vi "simulation analysis.vi"() -> ()   [LabVIEW 2009]
uses:
  subVIs/simulate (multiple).vi
  <vilib>/Utility/file.llb/Read From Spreadsheet File (I64).vi
  <vilib>/Analysis/NI_AALBase.lvlib
panel:
  out "y axis 2":dbl
  out "x axis 2":dbl
  out "x axis":dbl
  out "y axis":dbl
  out "output cluster":cluster{dbl[], "Best Linear Fit":dbl[]}[](graph)
  out "matches":i16[][](array[numeric])
  in  "source data folder(s)":cluster{"file path":path, "depth":i32}[](array[cluster])
  in  "estimated team value data":path
  # "blue score"
  # "red score"
  # "est blue"
  # "est red"
  # "red"
  # "blue"
  # "3"
  # "1"
  # "2"
  # "3"
  # "1"
  # "2"
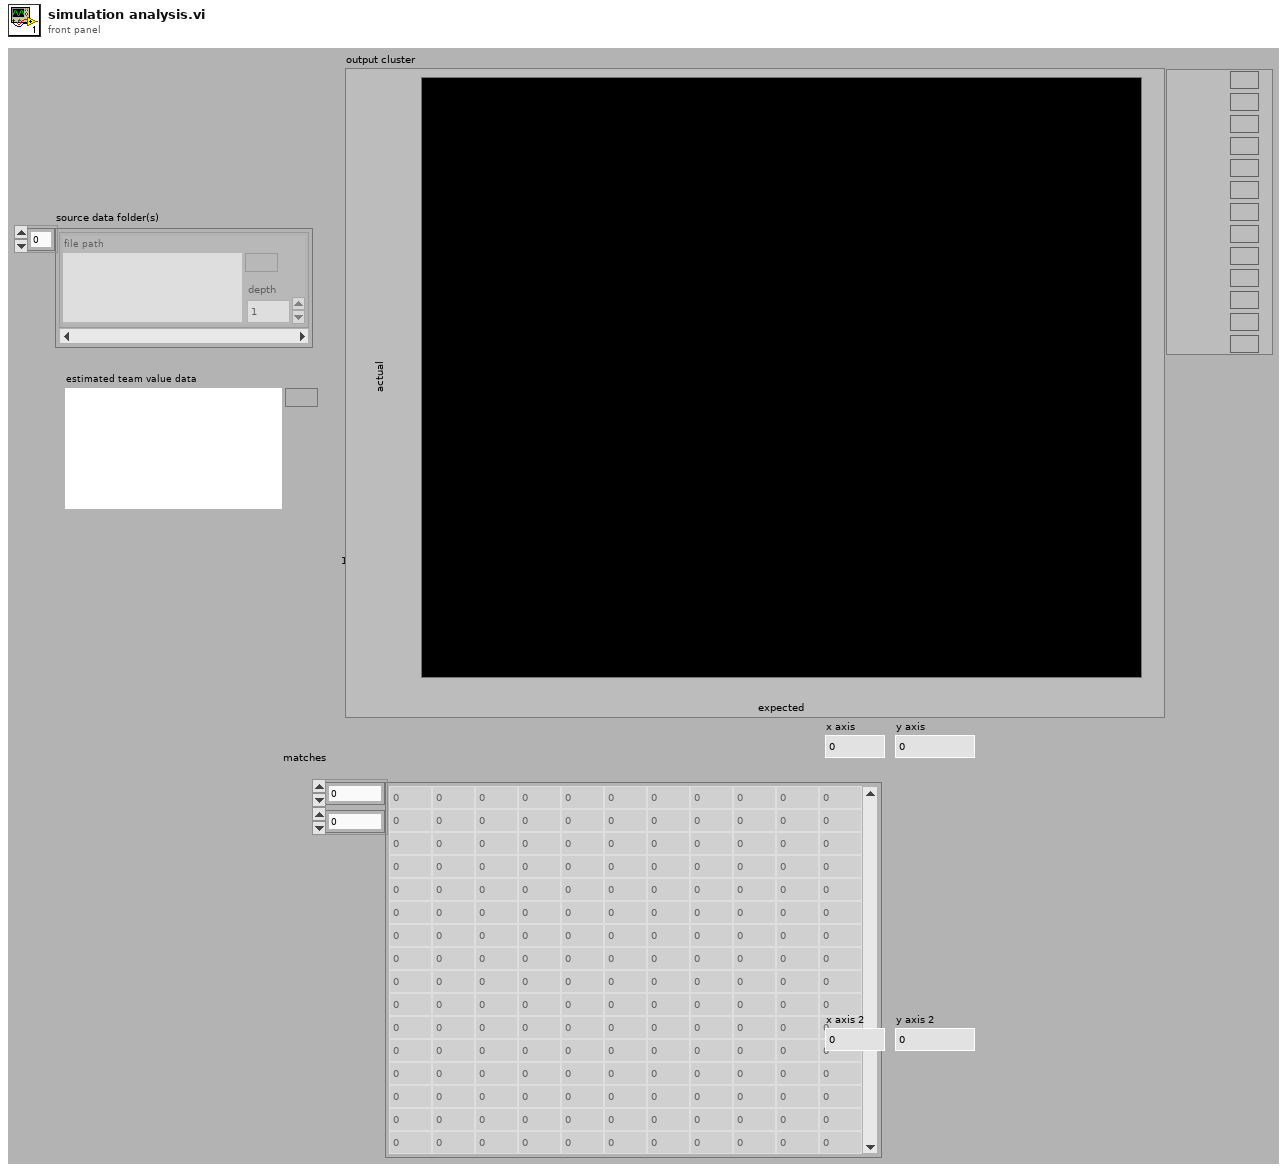
[diagram p1: front panel]
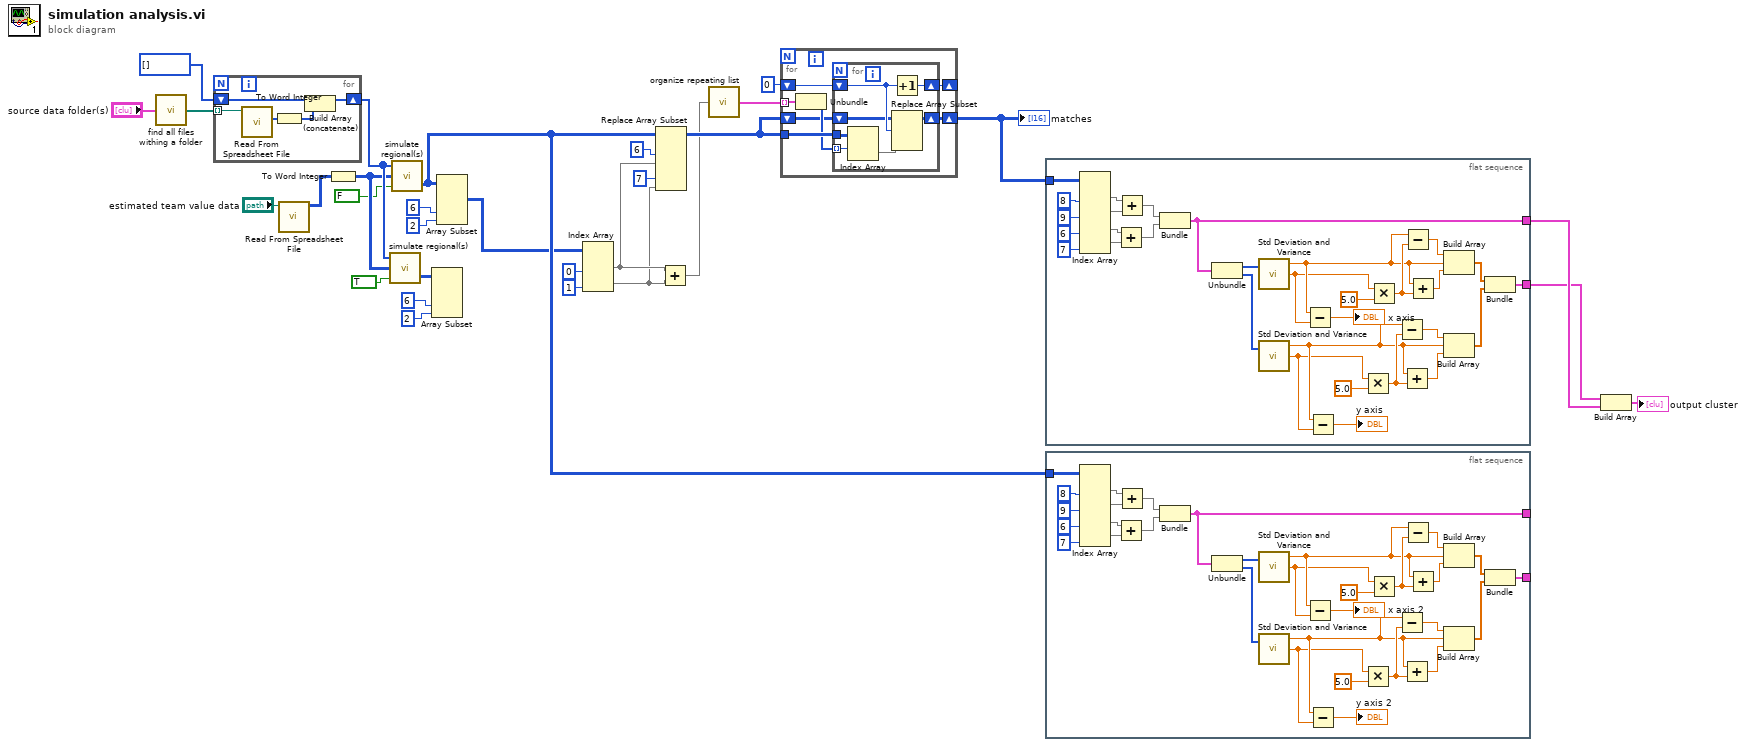
[diagram p0: block diagram]
diagram:
  n1 = call "find all files withing a folder.vi"("folders"="source data folder(s)") -> ("paths"=w28:path[])  [unwired: 1 out]
  n2 = for {
    shift-right: [w33] -> w21
    shift-left: i16[] [] -> [w31]
    tunnel: w28 -> [w34] mode=indexing
    n3 = call-poly <vilib>:"Read From Spreadsheet File.vi"("file path (dialog if empty)"=w34) -> ("first row"=w35:i64[])  [unwired: 6 in, 4 out]
    n4 = To Word Integer(number=w35) -> (16bit integer=w32:i16[])
    n5 = Build Array (concatenate)(w31, w32) -> (w33:i16[])
  }
  n6 = call-poly <vilib>:"Read From Spreadsheet File.vi"("file path (dialog if empty)"="estimated team value data") -> ("all rows"=w23:i64[][])  [unwired: 6 in, 4 out]
  n7 = To Word Integer(number=w23) -> (16bit integer=w20:i16[][])
  n8 = call-poly "simulate regional(s).vi"("liability?  (benefit)"=TRUE, "estimated values"=w20, "source data"=w21) -> ("Array"=w13:i16[][])  [unwired: 1 out]
  n9 = call-poly "simulate regional(s).vi"("liability?  (benefit)"=FALSE, "estimated values"=w20, "source data"=w21) -> ("Array"=w5:i16[][])  [unwired: 1 out]
  n10 = Array Subset(array=w13, index (col)=6 ("disabled index (col)"), length (col)=2 ("disabled index (col)")) -> ()  [unwired: 2 in, 1 out]
  n11 = Array Subset(array=w5, index (col)=6 ("disabled index (col)"), length (col)=2 ("disabled index (col)")) -> (w1:i16[][])  [unwired: 2 in]
  n12 = Index Array(array=w1, index (col) #1=0 ("disabled index (col)"), index (col) #2=1 ("index (col)")) -> (element #1=w8:i16[], element #2=w7:i16[])  [unwired: 2 in]
  n13 = Replace Array Subset(array=w5, new element #1=w8, index (col) #1=6 ("disabled index (col)"), new element #2=w7, index (col) #2=7 ("index (col)")) -> (w18:i16[][])  [unwired: 2 in]
  n14 = Add(x=w8, y=w7) -> (x+y=w6:i16[])
  n15 = call "organize repeating list.vi"("Array in"=w6) -> ("Array out"=w27:cluster{i16, i32[]}[])
  n16 = for {
    tunnel: w27 -> [w42] mode=indexing
    tunnel: w18 -> [w41]
    shift-right: [w38] -> w24
    shift-left: w18 -> [w37]
    shift-right: [w36] -> _
    shift-left: 0 -> [w39]
    n17 = Unbundle(w42) -> (w40:i32[])  [unwired: 1 out]
    n18 = for {
      tunnel: w41 -> [w49]
      tunnel: w40 -> [w48] mode=indexing
      shift-right: [w47] -> w36
      shift-left: w39 -> [w45]
      shift-right: [w44] -> w38
      shift-left: w37 -> [w43]
      n19 = Index Array(array=w49, index (row)=w48) -> (element=w46:i16[])  [unwired: 1 in]
      n20 = Increment(x=w45) -> (x+1=w47:i32)
      n21 = Replace Array Subset(array=w43, new element=w46, index (row)=w45) -> (w44:i16[][])  [unwired: 1 in]
    }
  }
  "matches" <- w24
  n22 = flat-sequence {
    tunnel: w24 -> [w58]
    tunnel: [w51] -> w3
    tunnel: [w50] -> w2
    frame #0 {
      n23 = Index Array(array=w58, index (col) #1=8 ("disabled index (col)"), index (col) #2=9 ("disabled index (col)"), index (col) #3=6 ("disabled index (col)"), index (col) #4=7 ("disabled index (col)")) -> (element #1=w63:i16[], element #2=w64:i16[], element #3=w62:i16[], element #4=w61:i16[])  [unwired: 4 in]
      n24 = Add(x=w62, y=w61) -> (x+y=w59:i16[])
      n25 = Add(x=w63, y=w64) -> (x+y=w60:i16[])
      n26 = Bundle(w60, w59) -> (w51:cluster{i16[], i16[]})  [unwired: 1 in]
      n27 = Unbundle(w51) -> (w80:i16[], w79:i16[])
      n28 = call <vilib>:"Std Deviation and Variance.vi"("X"=w80) -> ("mean"=w57:dbl, "standard deviation"=w56:dbl)  [unwired: 1 in, 1 out]
      n29 = call <vilib>:"Std Deviation and Variance.vi"("X"=w79) -> ("mean"=w55:dbl, "standard deviation"=w54:dbl)  [unwired: 1 in, 1 out]
      n30 = Subtract(x=w57, y=w56) -> (x-y=→"x axis":dbl)
      n31 = Subtract(x=w55, y=w54) -> (x-y=→"y axis":dbl)
      n32 = Multiply(x=w54, y=5.0) -> (x*y=w76:dbl)
      n33 = Multiply(x=w56, y=5.0) -> (x*y=w73:dbl)
      n34 = Subtract(x=w55, y=w76) -> (x-y=w74:dbl)
      n35 = Add(x=w55, y=w76) -> (x+y=w75:dbl)
      n36 = Subtract(x=w57, y=w73) -> (x-y=w70:dbl)
      n37 = Add(x=w57, y=w73) -> (x+y=w72:dbl)
      n38 = Build Array(w70, w57, w72) -> (w78:dbl[])
      n39 = Build Array(w74, w55, w75) -> (w69:dbl[])
      n40 = Bundle(w78, w69) -> (w50:cluster{dbl[], dbl[]})  [unwired: 1 in]
    }
  }
  n41 = flat-sequence {
    tunnel: w5 -> [w89]
    tunnel: [w82] -> _
    tunnel: [w81] -> _
    frame #0 {
      n42 = Index Array(array=w89, index (col) #1=8 ("disabled index (col)"), index (col) #2=9 ("disabled index (col)"), index (col) #3=6 ("disabled index (col)"), index (col) #4=7 ("disabled index (col)")) -> (element #1=w94:i16[], element #2=w95:i16[], element #3=w93:i16[], element #4=w92:i16[])  [unwired: 4 in]
      n43 = Add(x=w93, y=w92) -> (x+y=w90:i16[])
      n44 = Add(x=w94, y=w95) -> (x+y=w91:i16[])
      n45 = Bundle(w91, w90) -> (w82:cluster{i16[], i16[]})  [unwired: 1 in]
      n46 = Unbundle(w82) -> (w111:i16[], w110:i16[])
      n47 = call <vilib>:"Std Deviation and Variance.vi"("X"=w111) -> ("mean"=w88:dbl, "standard deviation"=w87:dbl)  [unwired: 1 in, 1 out]
      n48 = call <vilib>:"Std Deviation and Variance.vi"("X"=w110) -> ("mean"=w86:dbl, "standard deviation"=w85:dbl)  [unwired: 1 in, 1 out]
      n49 = Subtract(x=w88, y=w87) -> (x-y=→"x axis 2":dbl)
      n50 = Subtract(x=w86, y=w85) -> (x-y=→"y axis 2":dbl)
      n51 = Multiply(x=w85, y=5.0) -> (x*y=w107:dbl)
      n52 = Multiply(x=w87, y=5.0) -> (x*y=w104:dbl)
      n53 = Subtract(x=w86, y=w107) -> (x-y=w105:dbl)
      n54 = Add(x=w86, y=w107) -> (x+y=w106:dbl)
      n55 = Subtract(x=w88, y=w104) -> (x-y=w101:dbl)
      n56 = Add(x=w88, y=w104) -> (x+y=w103:dbl)
      n57 = Build Array(w101, w88, w103) -> (w109:dbl[])
      n58 = Build Array(w105, w86, w106) -> (w100:dbl[])
      n59 = Bundle(w109, w100) -> (w81:cluster{dbl[], dbl[]})  [unwired: 1 in]
    }
  }
  n60 = Build Array(w2, w3) -> (→"output cluster":cluster{dbl[], dbl[]}[])
